vi "RunTime.vi"(4 "no. measurements":i32, 5 "Probing done - new estimation":bool, 6 "Flag":enum16{"Update timer info", "Reset timer"}(ring)) -> (0 "Fraction of run completed":dbl format="%.2f", 1 "Estimated Completion Time":string, 2 "Estimated total time":string, 3 "Time so far":string)   [LabVIEW 2019]
doc: "Provides current run time, and updating estimate of total run time.\nFlag: 0 update timer info, 1: reset all time info"
panel:
  out "hours":u32
  out "mins":u32
  out "secs":u32
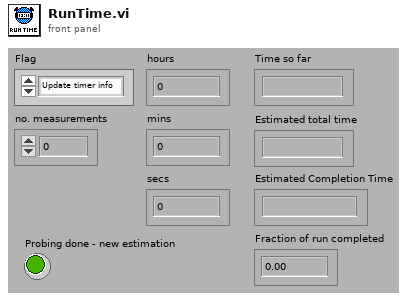
[diagram p1: front panel]
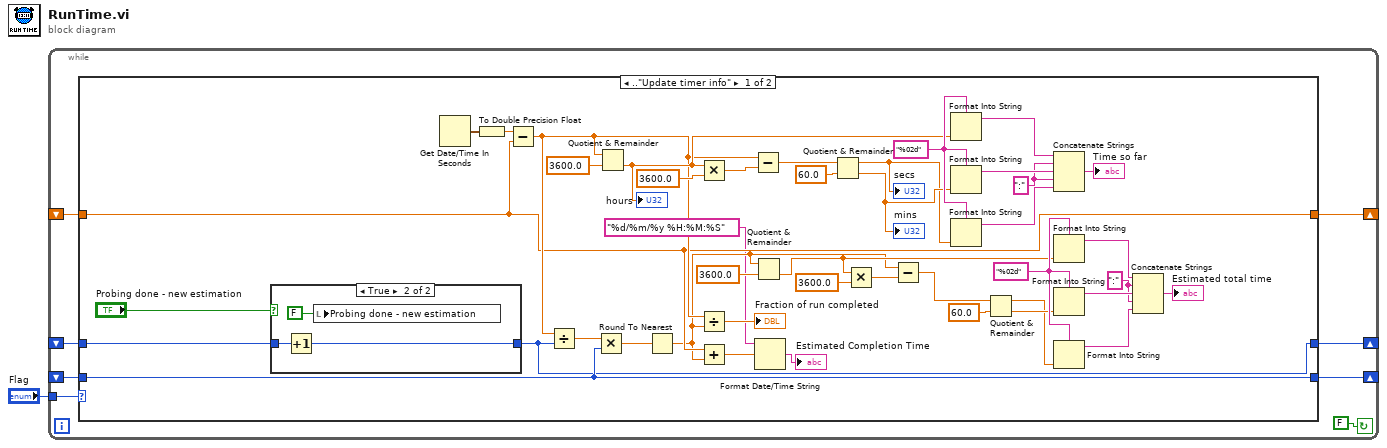
[diagram p0: block diagram]
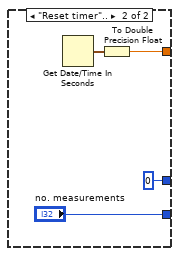
[diagram p3: hidden frame]
diagram:
  n1 = while {
    shift-right: [w7] -> _
    shift-left: _ -> [w8]
    tunnel: "Flag" -> [w9]
    shift-right: [w5] -> _
    shift-left: _ -> [w6]
    shift-right: [w3] -> _
    shift-left: _ -> [w4]
    stop <- FALSE continue-if-true
    n2 = case shown="..\"Update timer info\"" w9 {
      tunnel: w8 -> [w16 _]
      tunnel: [w16 w60] -> w7
      tunnel: w6 -> [w44 _]
      tunnel: [w40 0] -> w5
      tunnel: w4 -> [w42 _]
      tunnel: [w42 "no. measurements"] -> w3
      frame .."Update timer info" {
        w34 = ":"
        w37 = "%02d"
        w47 = ":"
        w50 = "%02d"
        n3 = case shown="True" "Probing done - new estimation" {
          tunnel: w44 -> [w53 w56]
          tunnel: [w53 w55] -> w40
          frame False {
          }
          frame True {
            n4 = Increment(x=w56) -> (x+1=w55:i32)
            n5 = local write "Probing done - new estimation"(FALSE) -> ()
          }
        }
        n6 = Get Date/Time In Seconds() -> (seconds since 1Jan1904=w11:timestamp)
        n7 = To Double Precision Float(number=w11) -> (double precision float=w52:dbl)
        n8 = Subtract(x=w52, y=w16) -> (x-y=w18:dbl)
        n9 = Divide(x=w18, y=w40) -> (x/y=w43:dbl)
        n10 = Multiply(x=w43, y=w42) -> (x*y=w41:dbl)
        n11 = Quotient & Remainder(x=w18, y=3600.0) -> (floor(x/y)=w20:dbl)  [unwired: 1 out]
        "hours" <- w20
        n12 = Round To Nearest(number=w41) -> (nearest integer value=w15:dbl)
        n13 = Multiply(x=w20, y=3600.0) -> (x*y=w22:dbl)
        n14 = Divide(x=w18, y=w15) -> (x/y=→"Fraction of run completed":dbl)
        n15 = Add(x=w16, y=w15) -> (x+y=w14:dbl)
        n16 = Subtract(x=w18, y=w22) -> (x-y=w21:dbl)
        n17 = Quotient & Remainder(x=w15, y=3600.0) -> (floor(x/y)=w25:dbl)  [unwired: 1 out]
        n18 = Format Date/Time String(time format string (%c)="%d/%m/%y %H:%M:%S", seconds (now)=w14) -> (date/time string=→"Estimated Completion Time":string)  [unwired: 1 in]
        n19 = Quotient & Remainder(x=w21, y=60.0) -> (x-y*floor(x/y)=w19:dbl, floor(x/y)=w39:dbl)
        "secs" <- w19
        "mins" <- w39
        n20 = Multiply(x=w25, y=3600.0) -> (x*y=w27:dbl)
        n21 = Subtract(x=w15, y=w27) -> (x-y=w26:dbl)
        n22 = Format Into String(format string=w50, w20) -> (resulting string=w49:string)  [unwired: 2 in, 1 out]
        n23 = Format Into String(format string=w50, w39) -> (resulting string=w48:string)  [unwired: 2 in, 1 out]
        n24 = Format Into String(format string=w50, w19) -> (resulting string=w46:string)  [unwired: 2 in, 1 out]
        n25 = Quotient & Remainder(x=w26, y=60.0) -> (x-y*floor(x/y)=w31:dbl, floor(x/y)=w32:dbl)
        n26 = Concatenate Strings(w49, w47, w48, w47, w46) -> (→"Time so far":string)
        n27 = Format Into String(format string=w37, w25) -> (resulting string=w36:string)  [unwired: 2 in, 1 out]
        n28 = Format Into String(format string=w37, w32) -> (resulting string=w35:string)  [unwired: 2 in, 1 out]
        n29 = Format Into String(format string=w37, w31) -> (resulting string=w33:string)  [unwired: 2 in, 1 out]
        n30 = Concatenate Strings(w36, w34, w35, w34, w33) -> (→"Estimated total time":string)
      }
      frame "Reset timer".. {
        n31 = Get Date/Time In Seconds() -> (seconds since 1Jan1904=w57:timestamp)
        n32 = To Double Precision Float(number=w57) -> (double precision float=w60:dbl)
      }
    }
  }
